vi "delay - four track.vi"(7 "Track Controls":T4 {"Track 3"."Volume Settings"."Volume" scale=1.0..10.0; "Track 3"."Volume Settings"."Pan" scale=0.0..1.0; "Track 3"."Effects Settings"."Delay 2" scale=0.0..10.0; "Track 3"."Effects Settings"."Delay" scale=0.0..1.0; "Track 2"."Volume Settings"."Volume" scale=1.0..10.0; "Track 2"."Volume Settings"."Pan" scale=0.0..1.0; "Track 2"."Effects Settings"."Delay 2" scale=0.0..10.0; "Track 2"."Effects Settings"."Delay" scale=0.0..1.0; "Track 1"."Volume Settings"."Volume" scale=1.0..10.0; "Track 1"."Volume Settings"."Pan" scale=0.0..1.0; "Track 1"."Effects Settings"."Delay 2" scale=0.0..10.0; "Track 1"."Effects Settings"."Delay" scale=0.0..1.0; "Track 0"."Volume Settings"."Volume" scale=1.0..10.0; "Track 0"."Volume Settings"."Pan" scale=0.0..1.0; "Track 0"."Effects Settings"."Delay 2" scale=0.0..10.0; "Track 0"."Effects Settings"."Delay" scale=0.0..1.0}, 10 "4-Track Audio in":T1, 11 "Delay Settings":T3 {"Wet/Dry" scale=0.0..5.0}) -> (3 "4-Track Audio out":T1)   [LabVIEW 2014]
uses:
  Controls/Track Controls.ctl
  Controls/Track Settings.ctl
  Controls/Track Effects Settings.ctl
  Controls/Track Volume Settings.ctl
  Controls/4 Track Audio.ctl
  Controls/Audio In.ctl
  Controls/Delay Controls.ctl
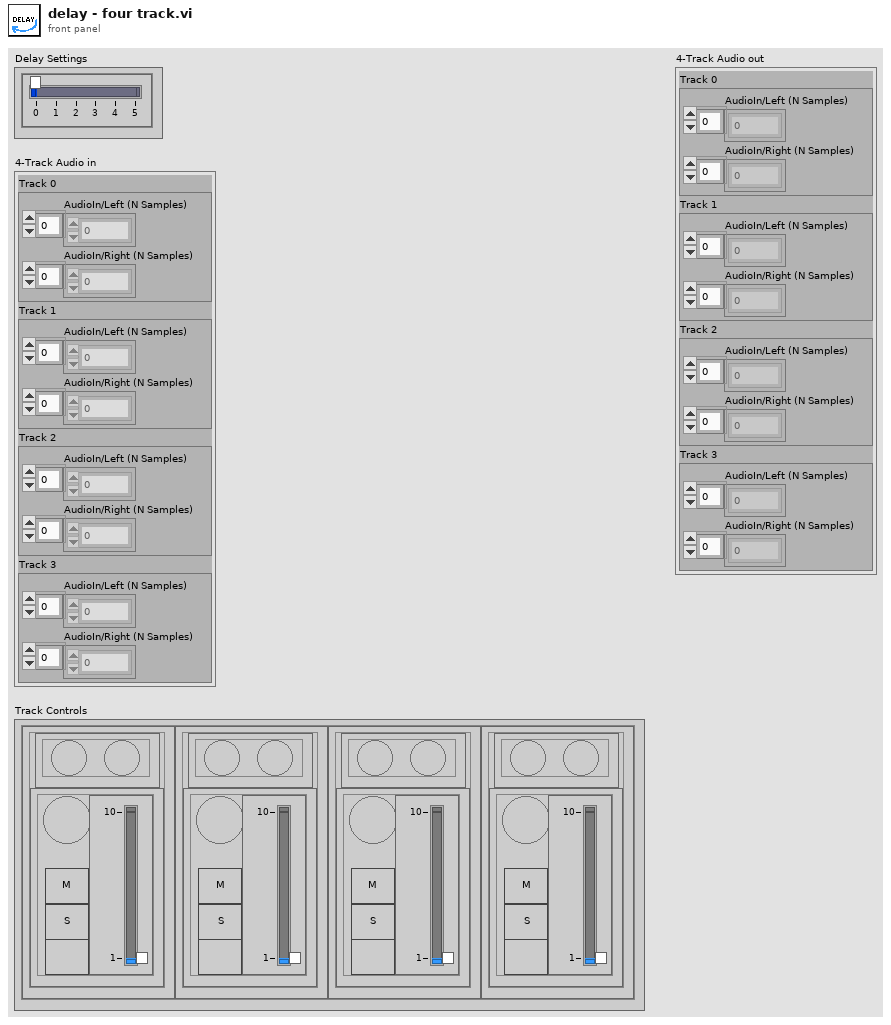
[diagram p1: front panel]
types:
  T1 = typedef "4 Track Audio.ctl" = cluster{"Track 0":T2, "Track 1":T2, "Track 2":T2, "Track 3":T2}
  T2 = typedef "Audio In.ctl" = cluster{"AudioIn/Left (N Samples)":i16[], "AudioIn/Right (N Samples)":i16[]}
  T3 = typedef "Delay Controls.ctl" = cluster{"Wet/Dry":u8}
  T4 = typedef "Track Controls.ctl" = cluster{"Track 0":T5, "Track 1":T5, "Track 2":T5, "Track 3":T5}
  T5 = typedef "Track Settings.ctl" = cluster{"Effects Settings":T6, "Volume Settings":T7}
  T6 = typedef "Track Effects Settings.ctl" = cluster{"Delay":dbl, "Delay 2":dbl}
  T7 = typedef "Track Volume Settings.ctl" = cluster{"Mute":bool, "Solo":bool, "Record":bool, "Pan":dbl, "Volume":dbl}
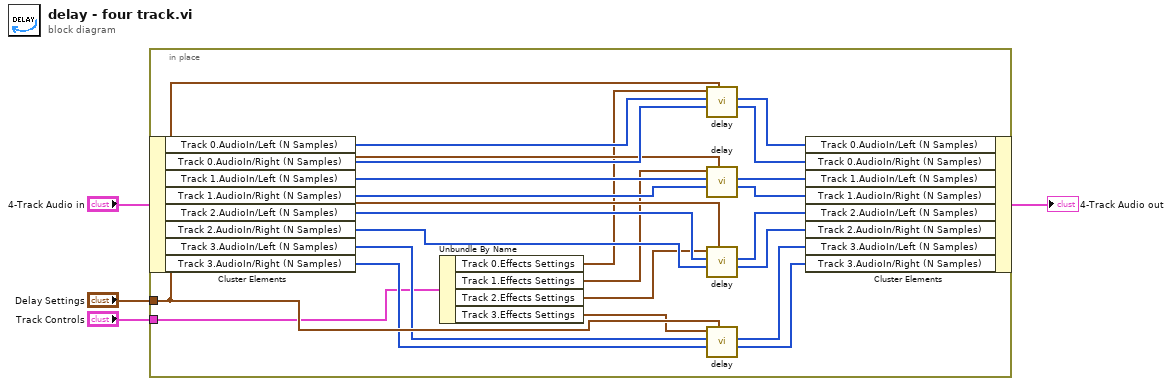
[diagram p0: block diagram]
diagram:
  n1 = in-place {
    in-place-border: "Delay Settings" -> [w14]
    in-place-border: "Track Controls" -> [w8]
    n2 = in-place-cluster #1("4-Track Audio in") -> ("Track 0.AudioIn/Left (N Samples)"=w26:i16[], "Track 0.AudioIn/Right (N Samples)"=w25:i16[], "Track 1.AudioIn/Left (N Samples)"=w22:i16[], "Track 1.AudioIn/Right (N Samples)"=w21:i16[], "Track 2.AudioIn/Left (N Samples)"=w18:i16[], "Track 2.AudioIn/Right (N Samples)"=w17:i16[], "Track 3.AudioIn/Left (N Samples)"=w13:i16[], "Track 3.AudioIn/Right (N Samples)"=w12:i16[])
    n3 = Unbundle By Name(w8) -> ("Track 0.Effects Settings"=w9:T6, "Track 1.Effects Settings"=w7:T6, "Track 2.Effects Settings"=w6:T6, "Track 3.Effects Settings"=w5:T6)
    n4 = call "delay.vi"("Delay Settings"=w14, "Audio R In"=w25, "Audio L In"=w26, "Effects"=w9) -> ("Audio R Out"=w23:i16[], "Audio L Out"=w24:i16[])  [unwired: 6 in]
    n5 = call "delay.vi"("Delay Settings"=w14, "Audio R In"=w21, "Audio L In"=w22, "Effects"=w7) -> ("Audio R Out"=w19:i16[], "Audio L Out"=w20:i16[])  [unwired: 6 in]
    n6 = call "delay.vi"("Delay Settings"=w14, "Audio R In"=w17, "Audio L In"=w18, "Effects"=w6) -> ("Audio R Out"=w15:i16[], "Audio L Out"=w16:i16[])  [unwired: 6 in]
    n7 = call "delay.vi"("Delay Settings"=w14, "Audio R In"=w12, "Audio L In"=w13, "Effects"=w5) -> ("Audio R Out"=w10:i16[], "Audio L Out"=w11:i16[])  [unwired: 6 in]
    n8 = in-place-cluster #1("Track 0.AudioIn/Left (N Samples)"=w24, "Track 0.AudioIn/Right (N Samples)"=w23, "Track 1.AudioIn/Left (N Samples)"=w20, "Track 1.AudioIn/Right (N Samples)"=w19, "Track 2.AudioIn/Left (N Samples)"=w16, "Track 2.AudioIn/Right (N Samples)"=w15, "Track 3.AudioIn/Left (N Samples)"=w11, "Track 3.AudioIn/Right (N Samples)"=w10) -> (→"4-Track Audio out":T1)
  }
